vi "UART_Close.vi"(3 "error in (no error)":errorcluster, 5 "VISA Resource In":refnum<visa-resource-name>) -> (0 "error out":errorcluster)   [LabVIEW 2015]
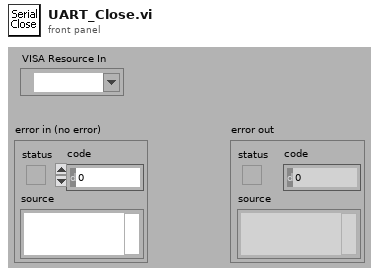
[diagram p1: front panel]
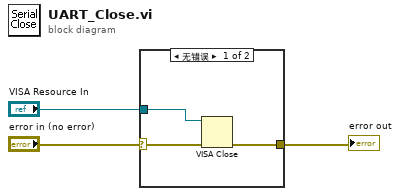
[diagram p0: block diagram]
diagram:
  n1 = case shown="无错误" "error in (no error)" {
    selector: "error in (no error)" -> [w4 w7]
    tunnel: [w6 w7] -> w3
    tunnel: "VISA Resource In" -> [w5 _]
    frame No Error {
      n2 = VISA Close(VISA resource name=w5, error in (no error)=w4) -> (error out=w6:errorcluster)
    }
    frame Error {
    }
  }
  "error out" <- w3
